vi "Lock.vi"(8 "error in (no error)":errorcluster, 11 "Timed Door in":refnum<class "Timed Door.lvclass">) -> (0 "error out":errorcluster, 3 "Timed Door out":refnum<class "Timed Door.lvclass">)   [LabVIEW 2018, in "Timed Door.lvclass"]
uses:
  Timed Door.lvclass
  Timed Door.lvclass/Timed Door.ctl
  Get Door.vi
  Set Door.vi
  Get Alarm DVR.vi
  Door/Door.lvclass
  Alarm/Alarm.lvclass
  Timer/Timer.lvclass
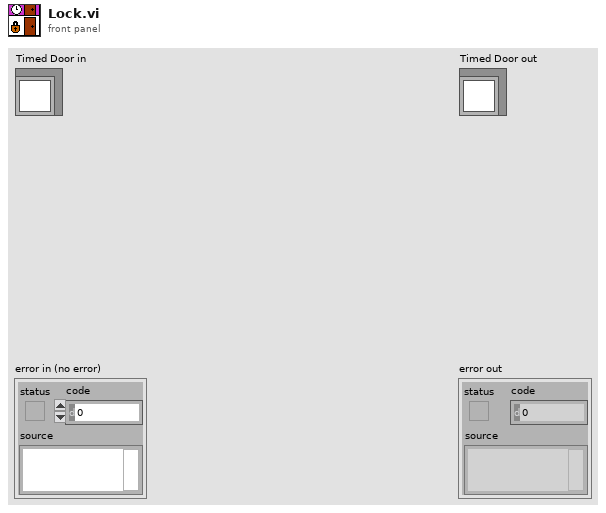
[diagram p1: front panel]
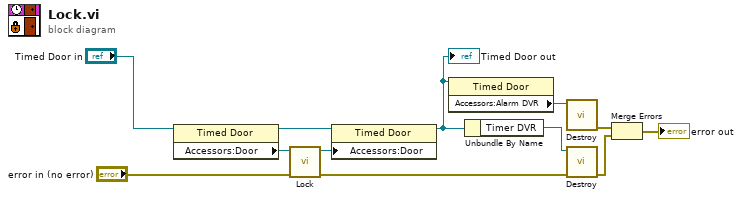
[diagram p0: block diagram]
diagram:
  n1 = property class="Timed Door"(reference="Timed Door in") -> (reference out=w5:refnum<class "Timed Door.lvclass">, "Accessors:Door"=w2:refnum<class "Door.lvclass">)  [unwired: 1 in, 1 out]
  n2 = call-dynamic "Lock.vi"("error in (no error)"="error in (no error)", "Door in"=w2) -> ("error out"=w11:errorcluster, "Door out"=w1:refnum<class "Door.lvclass">)  [unwired: 8 in]
  n3 = property class="Timed Door"(reference=w5, "Accessors:Door"=w1) -> (reference out=w3:refnum<class "Timed Door.lvclass">)  [unwired: 1 in, 1 out]
  "Timed Door out" <- w3
  n4 = property class="Timed Door"(reference=w3) -> ("Accessors:Alarm DVR"=w8:refnum<data-value>)  [unwired: 1 in, 2 out]
  n5 = Unbundle By Name(w3) -> ("Timer DVR"=w9:refnum<data-value>)
  n6 = call "Destroy.vi"("Alarm DVR"=w8) -> ("error out"=w6:errorcluster)  [unwired: 10 in]
  n7 = call "Destroy.vi"("error in (no error)"=w11, "Timer DVR"=w9) -> ("error out"=w10:errorcluster)  [unwired: 9 in]
  n8 = Merge Errors(w6, w10) -> (→"error out":errorcluster)
